vi "RSZVB Configure Mechanical Length.vi"(6 "Mechanical Length (0.0 m)":dbl format="%^.3e", 7 "Permittivity (1.00062 m)":dbl=1.00062 format="%^.3e", 8 "error in (no error)":errorcluster {"code" format="%.0x"}, 9 "Port (1)":i32=1, 10 "Channel (1)":i32=1, 11 "VISA session":refnum<visa-resource-name>) -> (0 "error out":errorcluster {"code" format="%.0x"}, 3 "dup VISA session":refnum<visa-resource-name>)   [LabVIEW 2011]
doc: "This VI configures parameters of mechanical length.\n\nNote(s):\n\nRemote-control command(s):\n[SENSe<Ch>:]CORRection:EDELay<port_no>:DISTance\n[SENSe<Ch>:]CORRection:EDELay<port_no>:DIELectric"
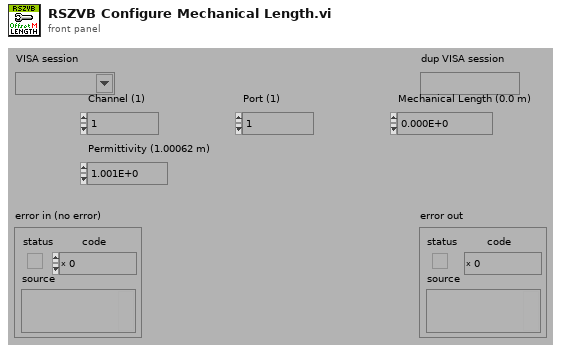
[diagram p1: front panel]
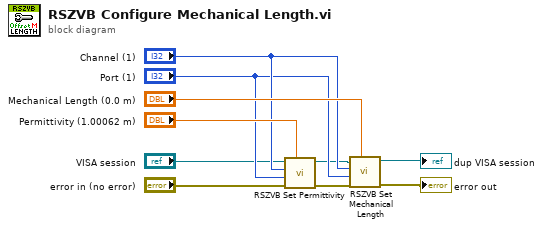
[diagram p0: block diagram]
diagram:
  n1 = call "RSZVB Set Permittivity.vi"("Permittivity (1.00062 m)"="Permittivity (1.00062 m)", "error in (no error)"="error in (no error)", "Port (1)"="Port (1)", "Channel (1)"="Channel (1)", "VISA session"="VISA session") -> ("error out"=w3:errorcluster, "dup VISA session"=w4:refnum<visa-resource-name>)  [unwired: 5 in]
  n2 = call "RSZVB Set Mechanical Length.vi"("Mechanical Length (0.0 m)"="Mechanical Length (0.0 m)", "error in (no error)"=w3, "Port (1)"="Port (1)", "Channel (1)"="Channel (1)", "VISA session"=w4) -> ("error out"=→"error out":errorcluster, "dup VISA session"=→"dup VISA session":refnum<visa-resource-name>)  [unwired: 5 in]
